vi "Single-Carrier Modulation.vi"(7 "QAM Comparison":enum16{"MT Modulate", "Homebrew"}(ring), 8 "Sampling Rate":i32=10, 9 "frequency":dbl=1.0 format="%0.2p", 10 "DataLen":i32=512, 11 "QAM Complexity":T2(ring)) -> (1 "sampling info":cluster{"Fs":dbl, "#s":dbl}={"Fs"=1000.0, "#s"=1000.0} {"Fs" format="%.2p"}, 3 "waveform":waveform(cdb))   [LabVIEW 2018]
uses:
  <vilib>/measure/maspectr.llb/FFT Spectrum (Real-Im) for 1 Chan (CDB).vi
  <vilib>/measure/NI_MAPro.lvlib
  <vilib>/measure/NI_MABase.lvlib
panel:
  out "#s":dbl
  out "FFT Plot (Imaginary)":dbl[](graph)
  out "Constellation Graph":T1(graph)
  out "FFT Plot (Real)":waveform(dbl)(graph)
  out "Waveform Graph":cluster{"f0":dbl, "df":dbl, "real part":dbl[]}(graph)
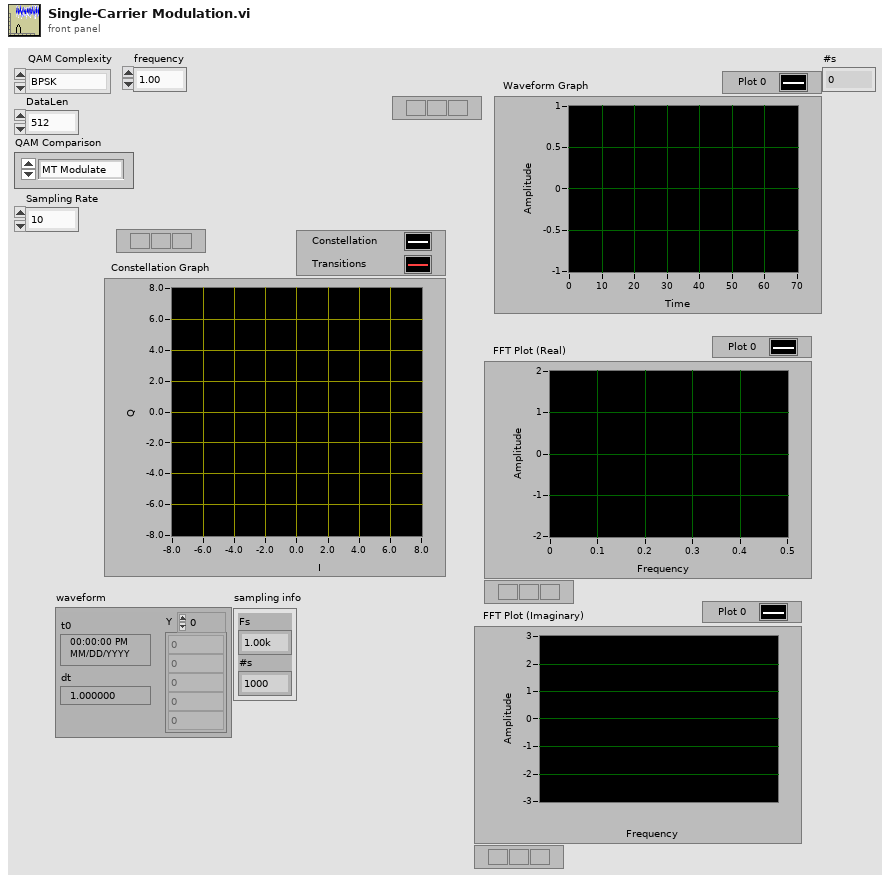
[diagram p1: front panel]
types:
  T1 = cluster{"Decimated Array":dbl[], "Decimated Array":dbl[]}[]
  T2 = enum16{"BPSK", "QPSK", "16-QAM", "64-QAM", "256-QAM"}
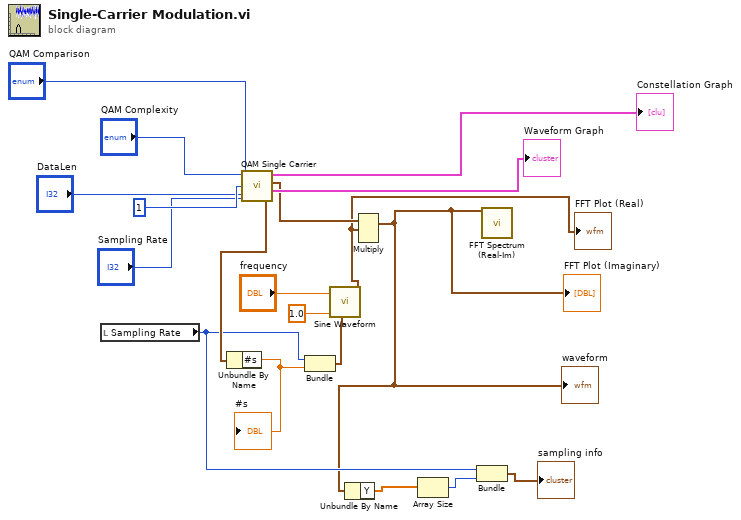
[diagram p0: block diagram]
diagram:
  n1 = local read "Sampling Rate"() -> (w7:i32)
  n2 = call "QAM Single Carrier.vi"("Symbol Rate"=1, "Samples/Symbol"="Sampling Rate", "DataLen"="DataLen", "QAM Comparison"="QAM Comparison", "QAM Complexity"="QAM Complexity") -> ("sampling info"=w12:cluster{"Fs":dbl, "#s":dbl}, "Waveform Graph"=→"Waveform Graph":cluster{"t0":dbl, "dt":dbl, "Y":dbl[]}, "Waveform"=w4:waveform(cdb), "Constellation Graph"=→"Constellation Graph":T1)
  n3 = Unbundle By Name(w12) -> ("#s"=w11:dbl)
  "#s" <- w11
  n4 = Bundle("Sampling Rate"=w7, "#s"=w11) -> (w8:cluster{"Sampling Rate":i32, "#s":dbl})  [unwired: 1 in]
  n5 = call <vilib>:"Sine Waveform.vi"("sampling info"=w8, "amplitude"=1.0, "frequency"="frequency") -> ("signal out"=w3:waveform(dbl))  [unwired: 7 in, 1 out]
  "FFT Plot (Real)" <- w3
  n6 = Multiply(1:w3, 2:w4) -> (0:w1:waveform(cdb))  [unwired: 1 in, 1 out]
  "FFT Plot (Imaginary)" <- w1
  "waveform" <- w1
  n7 = Unbundle By Name(w1) -> ("Y"=w2:cdb[])
  n8 = Array Size(array=w2) -> (size(s)=w6:i32)
  n9 = Bundle("Sampling Rate"=w7, w6) -> (→"sampling info":cluster{"Sampling Rate":i32, i32})  [unwired: 1 in]
  n10 = call-poly <vilib>:"FFT Spectrum (Real-Im).vi"("time signal"=w1) -> ()  [unwired: 6 in, 5 out]
